vi "ep_Torque Check Error (1 Motor with IC).vi"(0 "phase voltage waveforms":waveform(dbl)[](array[waveform]), 1 "current waveforms":waveform(dbl)[](array[waveform]), 5 "error in (no error)":errorcluster, 6 "fundamental frequency [Hz]":dbl=50.0, 8 "reset? (F)":bool) -> (19 "error out":errorcluster)   [LabVIEW 2014, in "NI_EP_Motor Monitoring.lvlib"]
uses:
  <vilib>/addons/Electrical Power/Motor Monitoring/NI_EP_Motor Monitoring.lvlib
  <vilib>/addons/Electrical Power/Power Measurement/NI_EP_Power Measurement.lvlib
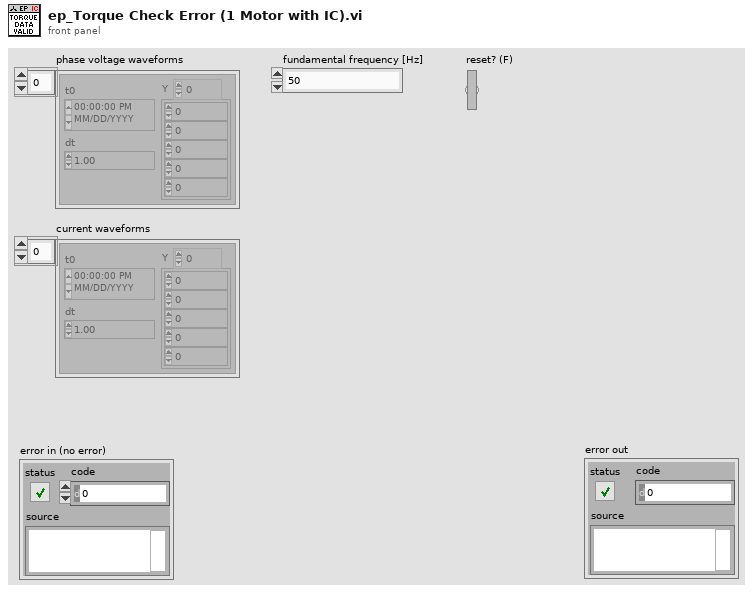
[diagram p1: front panel]
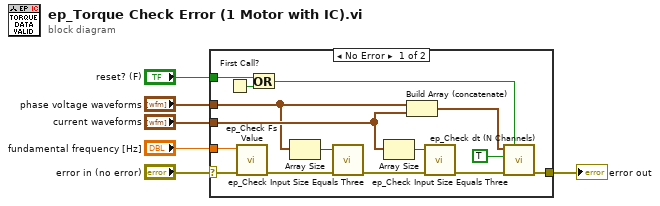
[diagram p0: block diagram]
diagram:
  n1 = case shown="No Error" "error in (no error)" {
    selector: "error in (no error)" -> [w21 w22]
    tunnel: "fundamental frequency [Hz]" -> [w20 _]
    tunnel: "phase voltage waveforms" -> [w8 _]
    tunnel: "current waveforms" -> [w10 _]
    tunnel: "reset? (F)" -> [w16 _]
    tunnel: [w14 w22] -> w1
    frame No Error {
      n2 = First Call?() -> (First Call?: T/F=w17:bool)
      n3 = call <vilib>:"ep_Check Fs Value.vi"("error in (no error)"=w21, "fundamental frequency [Hz]"=w20) -> ("error out"=w13:errorcluster)  [unwired: 9 in]
      n4 = Or(x=w16, y=w17) -> (x .or. y?=w15:bool)
      n5 = Array Size(array=w8) -> (size(s)=w9:i32)
      n6 = call <vilib>:"ep_Check Input Size Equals Three.vi"("error in (no error)"=w13, "# of channels"=w9) -> ("error out"=w12:errorcluster)  [unwired: 9 in]
      n7 = Array Size(array=w10) -> (size(s)=w11:i32)
      n8 = Build Array (concatenate)(w8, w10) -> (w19:waveform(dbl)[])
      n9 = call <vilib>:"ep_Check Input Size Equals Three.vi"("error in (no error)"=w12, "# of channels"=w11) -> ("error out"=w7:errorcluster)  [unwired: 9 in]
      n10 = call <vilib>:"ep_Check dt (N Channels).vi"("reset? (F)"=w15, "error in (no error)"=w7, "waveforms only? (F)"=TRUE, "waveforms"=w19) -> ("error out"=w14:errorcluster)  [unwired: 3 in, 4 out]
    }
    frame Error {
    }
  }
  "error out" <- w1
